vi "PC_NS_Signal connect_communication.vi"(7 "Maximum Reader":i32=20, 8 "error in (no error)":errorcluster, 11 "PC_NS_Signal in":refnum<class "PC_NS_Signal.lvclass">) -> (0 "error out":errorcluster, 3 "PC_NS_Signal out":refnum<class "PC_NS_Signal.lvclass">)   [LabVIEW 2018, in "PC_NS_Signal.lvclass"]
uses:
  PC_NS_Signal.lvclass
  PC_NS_Signal.lvclass/PC_NS_Signal.ctl
  <resource>/objmgr/ni.var.rc
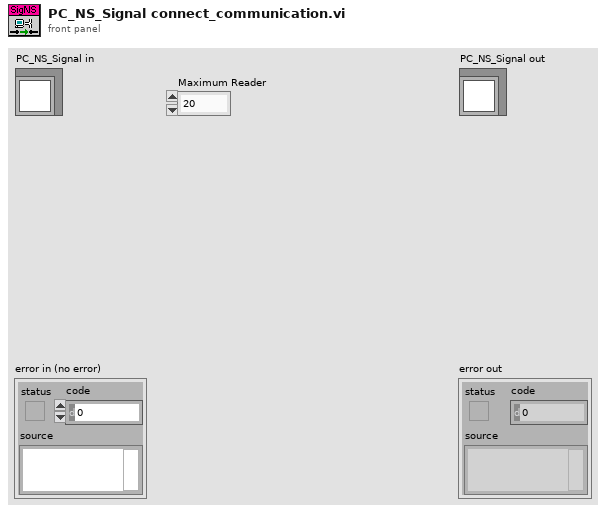
[diagram p1: front panel]
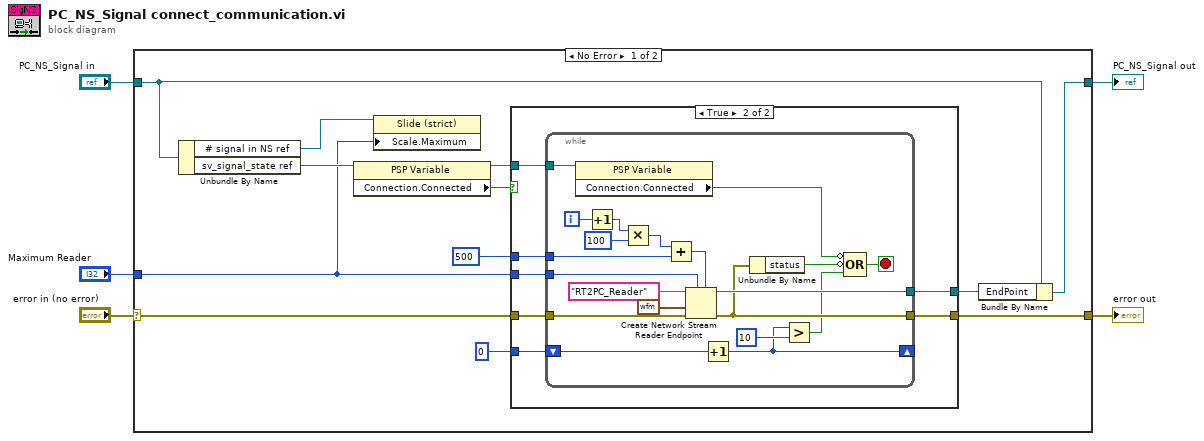
[diagram p0: block diagram]
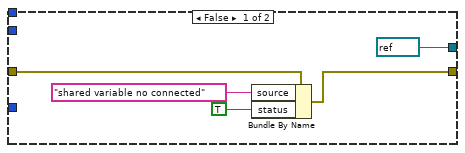
[diagram p2: hidden frame]
diagram:
  n1 = case shown="No Error" "error in (no error)" {
    selector: "error in (no error)" -> [w11 w51]
    tunnel: [w12 w51] -> w4
    tunnel: [w16 w50] -> w2
    tunnel: "PC_NS_Signal in" -> [w7 w50]
    tunnel: "Maximum Reader" -> [w9 _]
    frame No Error {
      n2 = Unbundle By Name(w7) -> ("# signal in NS ref"=w10:refnum<vi>, "sv_signal_state ref"=w15:refnum<k21>)
      n3 = property class="PSP Variable"(reference=w15) -> (reference out=w13:refnum<k21>, "Connection.Connected"=w14:bool)  [unwired: 1 in, 1 out]
      n4 = property class="Slide (strict)"(reference=w10, "Scale.Maximum"=w9) -> ()  [unwired: 1 in, 2 out]
      n5 = case shown="True" w14 {
        tunnel: [w18 w26] -> w12
        tunnel: [refnum<k21> refnum ("EndPoint") w29] -> w17
        tunnel: w11 -> [w19 w28]
        tunnel: w9 -> [_ w27]
        tunnel: w13 -> [_ w25]
        tunnel: 0 -> [_ w24]
        tunnel: 500 -> [_ w23]
        frame False {
          n6 = Bundle By Name(cluster=w19, "source"="shared variable no connected", "status"=TRUE) -> (w18:errorcluster)
        }
        frame True {
          n7 = while {
            tunnel: [w47] -> w29
            tunnel: w27 -> [w45]
            tunnel: w28 -> [w46]
            tunnel: [w43] -> w26
            tunnel: w25 -> [w44]
            shift-right: [w39] -> _
            shift-left: w24 -> [w41]
            tunnel: w23 -> [w31]
            i -> [w35]
            stop <- w42 stop-if-true
            n8 = property class="PSP Variable"(reference=w44) -> ("Connection.Connected"=w37:bool)  [unwired: 1 in, 2 out]
            n9 = Increment(x=w35) -> (x+1=w33:i32)
            n10 = Multiply(x=w33, y=100) -> (x*y=w32:i32)
            n11 = Add(x=w32, y=w31) -> (x+y=w30:i32)
            n12 = Create Network Stream Reader Endpoint(5:w30, 7:w45, 8:w46, 9:waveform(i16) {"t0"=timestamp(0 s since 1904-01-01), "dt"=1.0, "Y"=[]} ("element"), 11:"RT2PC_Reader" ("EndPoint")) -> (0:w43:errorcluster, 3:w47:refnum<k21>)  [unwired: 2 in]
            n13 = Increment(x=w41) -> (x+1=w39:i32)
            n14 = Unbundle By Name(w43) -> ("status"=w36:bool)
            n15 = Greater?(x=w39, y=10) -> (0:w38:bool)
            n16 = Compound Arithmetic op=OR(invert w37, invert w36, w38) -> (w42:bool)
          }
        }
      }
      n17 = Bundle By Name(cluster=w7, "EndPoint"=w17) -> (w16:refnum<class "PC_NS_Signal.lvclass">)
    }
    frame Error {
    }
  }
  "error out" <- w4
  "PC_NS_Signal out" <- w2
